vi "Build JSON Array Elements Paths.vi"(10 "No Of Elements":i32, 11 "JSON Array Path":string) -> (3 "Paths":string[](array[string]))   [LabVIEW 2026, in "Template Deployment Hooks.lvlib"]
uses:
  Template Deployment Hooks.lvlib
  <vilib>/Utility/error.llb/whitespace.ctl
  <vilib>/Utility/error.llb/Trim Whitespace (string).vi
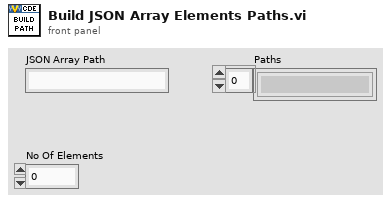
[diagram p1: front panel]
types:
  T1 = typedef "whitespace.ctl" = u16
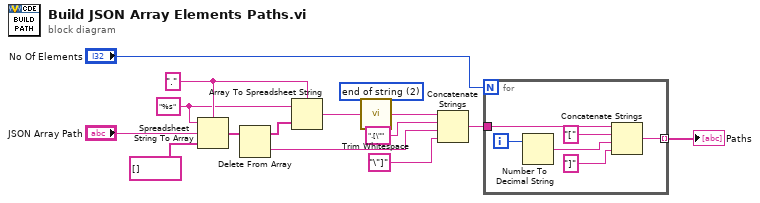
[diagram p0: block diagram]
diagram:
  w1 = T1 2 items=["both", "start of string", "end of string"] ("location (both)")
  w7 = "%s" ("format string")
  w9 = "." ("delimiter (Tab)")
  n1 = Spreadsheet String To Array(delimiter (Tab)=w9, format string=w7, spreadsheet string="JSON Array Path", array type (2D Dbl)=string[] []) -> (array=w11:string[])
  n2 = Delete From Array(array=w11) -> (deleted portion=w3:string, array with subset deleted=w8:string[])  [unwired: 2 in]
  n3 = Array To Spreadsheet String(delimiter (Tab)=w9, array=w8, 3:w7) -> (spreadsheet string=w6:string)
  n4 = call-poly <vilib>:"Trim Whitespace.vi"("string"=w6, "location (both)"=w1) -> ("trimmed string"=w2:string)
  n5 = Concatenate Strings(w2, ".[\"" ("string"), w3, "\"]" ("string")) -> (w13:string)
  n6 = for {
    N: "No Of Elements" -> [_]
    tunnel: w13 -> [w21]
    tunnel: [w16] -> w14 mode=indexing
    i -> [w18]
    n7 = Number To Decimal String(number=w18) -> (decimal integer string=w17:string)  [unwired: 1 in]
    n8 = Concatenate Strings(w21, "[" ("string"), w17, "]" ("string")) -> (w16:string)
  }
  "Paths" <- w14
